vi "Initialize Parameters.vi"(8 "error in (no error)":errorcluster, 11 "Hot And Cold Source Unit View in":refnum<class "Hot And Cold Source Unit View.lvclass">) -> (0 "error out":errorcluster, 3 "Hot And Cold Source Unit View out":refnum<class "Hot And Cold Source Unit View.lvclass">)   [LabVIEW 2013, in "Hot And Cold Source Unit View.lvlib" / "Hot And Cold Source Unit View.lvclass"]
uses:
  Hot And Cold Source Unit View.lvclass
  Hot And Cold Source Unit View.lvclass/Hot And Cold Source Unit View.ctl
  Common/Control Reference/Control Reference.lvlib
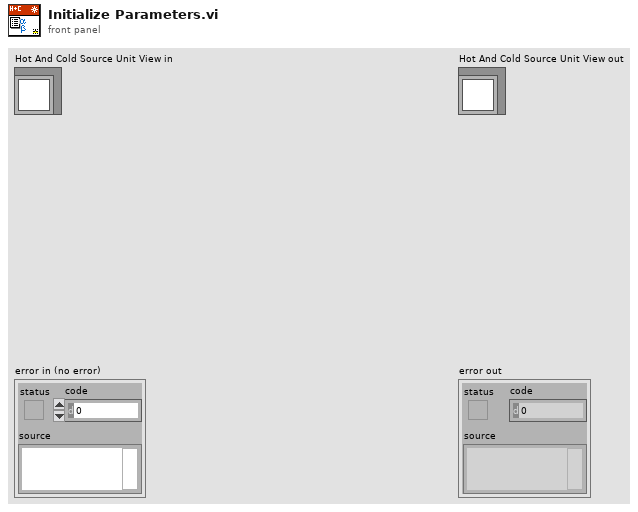
[diagram p1: front panel]
types:
  T1 = enum8{"Enabled", "Disabled", "Disabled and Grayed Out"}
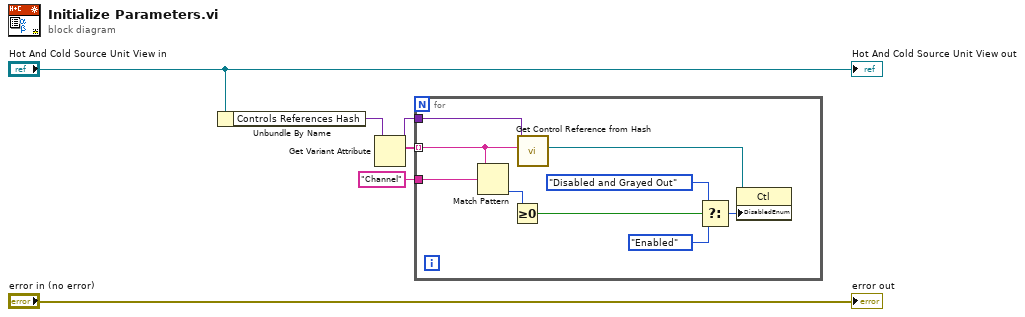
[diagram p0: block diagram]
diagram:
  n1 = Unbundle By Name("Hot And Cold Source Unit View in") -> ("Controls References Hash"=w4:variant)
  n2 = Get Variant Attribute(Variant=w4) -> (duplicate Variant=w3:variant, names=w5:string[])  [unwired: 3 in, 2 out]
  n3 = for {
    tunnel: w5 -> [w14] mode=indexing
    tunnel: w3 -> [w15]
    tunnel: "Channel" -> [w7]
    n4 = Match Pattern(string=w14, regular expression=w7) -> (offset past match=w12:i32)  [unwired: 1 in, 3 out]
    n5 = Greater Or Equal To 0?(x=w12) -> (x >= 0?=w11:bool)
    n6 = call "Get Control Reference from Hash.vi"("control label"=w14, "controls references hash"=w15) -> ("control reference"=w13:refnum<vi>)  [unwired: 6 in, 3 out]
    n7 = Select(t=T1."Disabled and Grayed Out" ("Disabled"), s=w11, f=T1."Enabled" ("Disabled")) -> (s? t:f=w8:T1)
    n8 = property class="Ctl"(reference=w13, "DisabledEnum"=w8) -> ()  [unwired: 1 in, 2 out]
  }
  "error out" <- "error in (no error)"
  "Hot And Cold Source Unit View out" <- "Hot And Cold Source Unit View in"
